vi "Config Load.vi"(8 "error in (no error)":errorcluster, 11 "Text":string) -> (0 "error out":errorcluster, 3 "Sections":T1(array[cluster]))   [LabVIEW 2018]
uses:
  <vilib>/regexp/Match Regular Expression.xnode
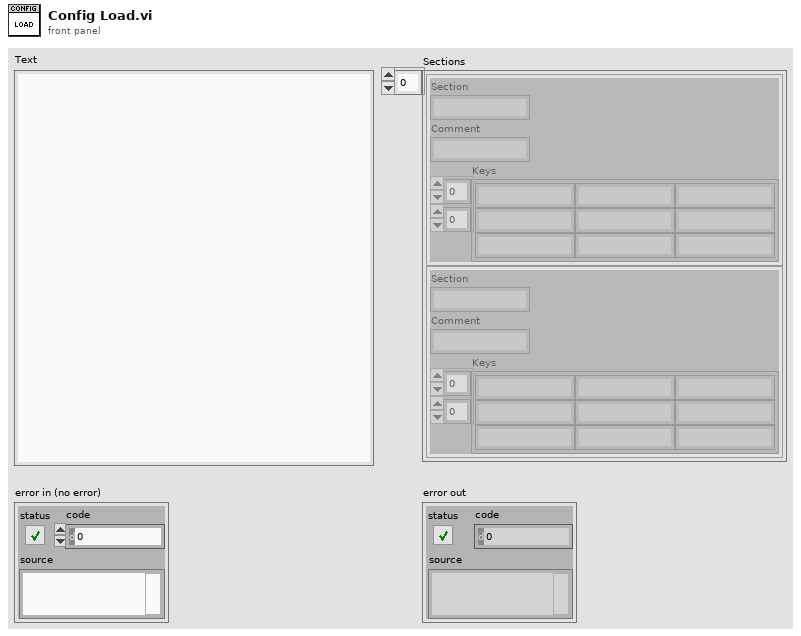
[diagram p1: front panel]
types:
  T1 = cluster{"Section":string, "Comment":string, "Keys":string[][]}[]
  T2 = cluster{"Section":string, "Comment":string, "Keys":string[][]}
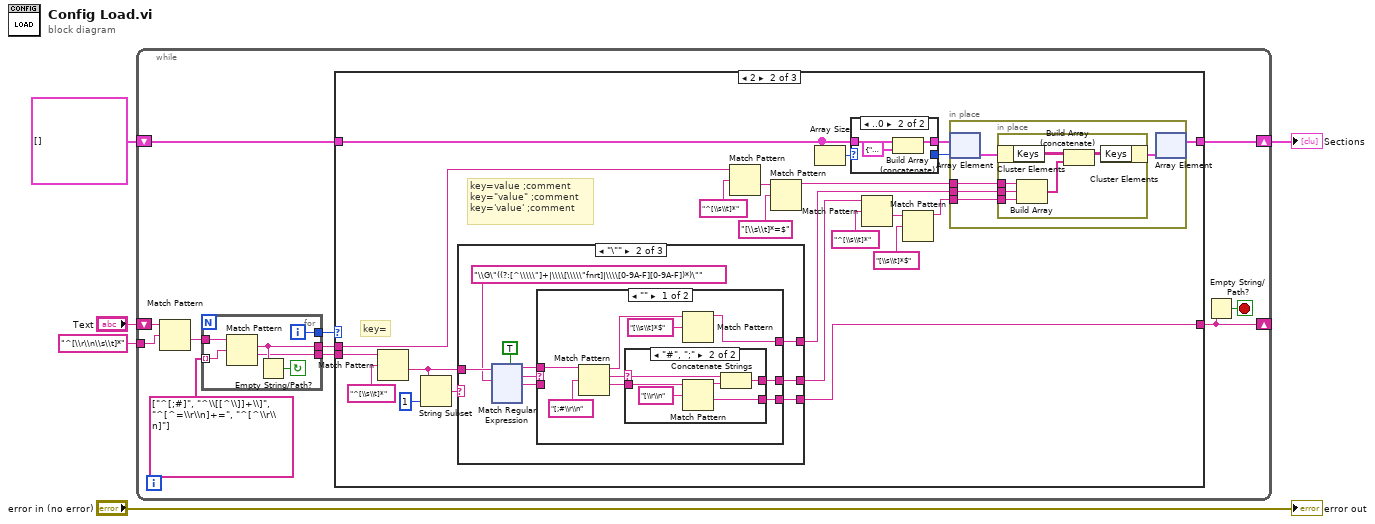
[diagram p0: block diagram]
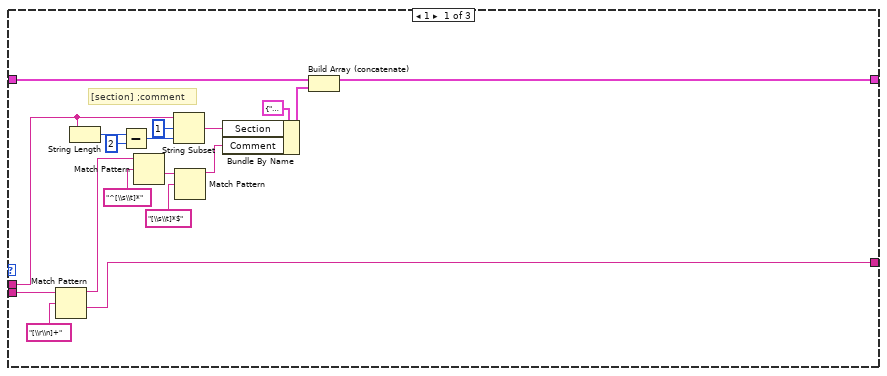
[diagram p2: hidden frame]
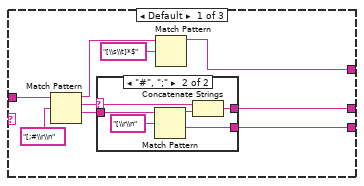
[diagram p3: hidden frame]
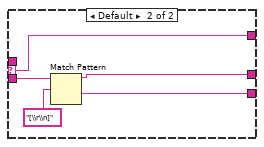
[diagram p6: hidden frame]
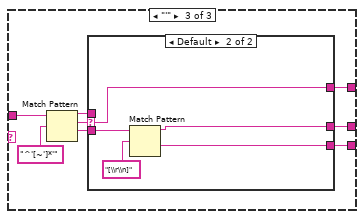
[diagram p7: hidden frame]
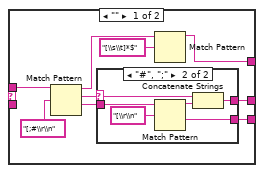
[diagram p8: hidden frame]
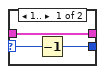
[diagram p10: hidden frame]
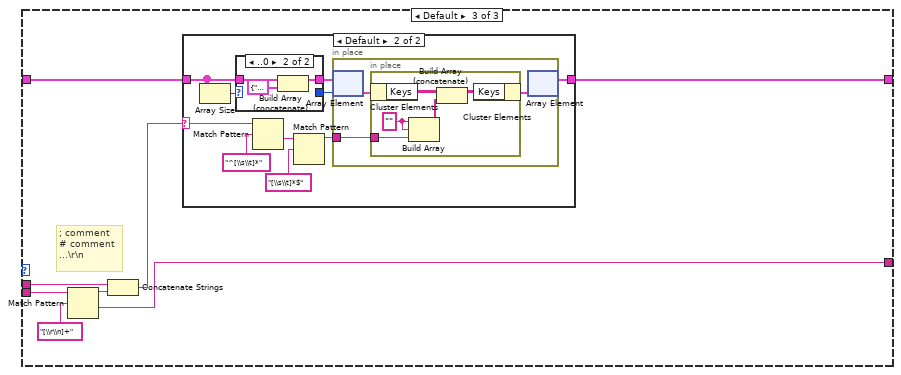
[diagram p11: hidden frame]
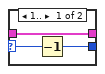
[diagram p13: hidden frame]
diagram:
  n1 = while {
    tunnel: "^[\\r\\n\\s\\t]*" ("regular expression") -> [w16]
    shift-right: [w9] -> _
    shift-left: "Text" -> [w15]
    shift-right: [w10] -> w1
    shift-left: T1 [] ("Sections") -> [w12]
    stop <- w8 stop-if-true
    n2 = Match Pattern(string=w15, regular expression=w16) -> (after substring=w14:string)  [unwired: 1 in, 3 out]
    n3 = for {
      tunnel: string[] ["^[;#]", "^\\[[^\\]]+\\]", "^[^=\\r\\n]+=", "^[^\\r\\n]"] -> [w304] mode=indexing
      tunnel: w14 -> [w303]
      tunnel: [w301] -> w7
      tunnel: [w300] -> w13
      tunnel: [w299] -> w11
      i -> [w300]
      stop <- w302 continue-if-true
      n4 = Match Pattern(string=w303, regular expression=w304) -> (match substring=w301:string, after substring=w299:string)  [unwired: 1 in, 2 out]
      n5 = Empty String/Path?(string/path=w301) -> (empty?=w302:bool)
    }
    n6 = case shown="2" w13 {
      tunnel: w12 -> [w21 w49 w273]
      tunnel: w11 -> [w18 w41 w269]
      tunnel: [w20 w48 w272] -> w10
      tunnel: [w17 w37 w268] -> w9
      tunnel: w7 -> [w19 w44 w266]
      frame 1 {
        # "[section] ;comment"
        n7 = Match Pattern(string=w18, regular expression="[\\r\\n]+") -> (before substring=w23:string, after substring=w17:string)  [unwired: 1 in, 2 out]
        n8 = String Length(string=w19) -> (length=w30:i32)
        n9 = Subtract(x=w30, y=2) -> (x-y=w28:i32)
        n10 = Match Pattern(string=w23, regular expression="^[\\s\\t]*") -> (after substring=w24:string)  [unwired: 1 in, 3 out]
        n11 = String Subset(string=w19, offset (0)=1, length (rest)=w28) -> (substring=w27:string)
        n12 = Match Pattern(string=w24, regular expression="[\\s\\t]*$") -> (before substring=w22:string)  [unwired: 1 in, 3 out]
        n13 = Bundle By Name(cluster=T2 {"Section"="", "Comment"="", "Keys"=[]} ("array"), "Section"=w27, "Comment"=w22) -> (w32:T2)
        n14 = Build Array (concatenate)(w21, w32) -> (w20:T1)
      }
      frame 2 {
        # "key=value ;comment\nkey=\"value\" ;comment\nkey='value' ;comment"
        # "key="
        n15 = Match Pattern(string=w41, regular expression="^[\\s\\t]*") -> (after substring=w38:string)  [unwired: 1 in, 3 out]
        n16 = String Subset(string=w38, length (rest)=1 ("length (rest)")) -> (substring=w39:string)  [unwired: 1 in]
        n17 = case shown="\"\\\"\"" w39 {
          tunnel: w38 -> [w64 w81 w224]
          tunnel: [w61 w74 w225] -> w37
          tunnel: [w60 w75 w226] -> w36
          tunnel: [w57 w78 w227] -> w35
          frame Default {
            n18 = Match Pattern(string=w64, regular expression="[;#\\r\\n") -> (before substring=w58:string, match substring=w62:string, after substring=w63:string)  [unwired: 1 in, 1 out]
            n19 = case shown="\"#\", \";\"" w62 {
              selector: w62 -> [_ w70]
              tunnel: w63 -> [w66 w71]
              tunnel: [w66 w68] -> w61
              tunnel: [_ w67] -> w60
              frame Default {
              }
              frame "#", ";" {
                n20 = Match Pattern(string=w71, regular expression="[\\r\\n") -> (before substring=w69:string, after substring=w68:string)  [unwired: 1 in, 2 out]
                n21 = Concatenate Strings(w70, w69) -> (w67:string)
              }
            }
            n22 = Match Pattern(string=w58, regular expression="[\\s\\t]*$") -> (before substring=w57:string)  [unwired: 1 in, 3 out]
          }
          frame "\"" {
            n23 = xnode "Match Regular Expression"("input string"=w81, "regular expression"="\\G\"((?:[^\\\\\"]+|\\\\[\\\\\"fnrt]|\\\\[0-9A-F][0-9A-F])*)\"", "multiline? (F)"=TRUE) -> ("before match"=w77:string, "whole match"=w79:string, "after match"=w76:string)  [unwired: 3 in, 2 out]
            n24 = case shown="\"\"" w79 {
              selector: w79 -> [_ w102]
              tunnel: [w82 w102] -> w78
              tunnel: w77 -> [w87 _]
              tunnel: w76 -> [_ w100]
              tunnel: [w86 w99] -> w75
              tunnel: [w85 w98] -> w74
              frame "" {
                n25 = Match Pattern(string=w87, regular expression="[;#\\r\\n") -> (before substring=w83:string, match substring=w88:string, after substring=w89:string)  [unwired: 1 in, 1 out]
                n26 = case shown="\"#\", \";\"" w88 {
                  selector: w88 -> [_ w95]
                  tunnel: w89 -> [w91 w96]
                  tunnel: [w91 w93] -> w85
                  tunnel: [_ w92] -> w86
                  frame Default {
                  }
                  frame "#", ";" {
                    n27 = Match Pattern(string=w96, regular expression="[\\r\\n") -> (before substring=w94:string, after substring=w93:string)  [unwired: 1 in, 2 out]
                    n28 = Concatenate Strings(w95, w94) -> (w92:string)
                  }
                }
                n29 = Match Pattern(string=w83, regular expression="[\\s\\t]*$") -> (before substring=w82:string)  [unwired: 1 in, 3 out]
              }
              frame Default {
                n30 = Match Pattern(string=w100, regular expression="[\\r\\n]") -> (before substring=w99:string, after substring=w98:string)  [unwired: 1 in, 2 out]
              }
            }
          }
          frame "'" {
            n31 = Match Pattern(string=w224, regular expression="^'[~']*'") -> (before substring=w223:string, match substring=w222:string, after substring=w221:string)  [unwired: 1 in, 1 out]
            n32 = case shown="Default" w222 {
              selector: w222 -> [_ w248]
              tunnel: [w228 w248] -> w227
              tunnel: w223 -> [w233 _]
              tunnel: w221 -> [_ w246]
              tunnel: [w232 w245] -> w226
              tunnel: [w231 w244] -> w225
              frame "" {
                n33 = Match Pattern(string=w233, regular expression="[;#\\r\\n") -> (before substring=w229:string, match substring=w234:string, after substring=w235:string)  [unwired: 1 in, 1 out]
                n34 = case shown="\"#\", \";\"" w234 {
                  selector: w234 -> [_ w241]
                  tunnel: w235 -> [w237 w242]
                  tunnel: [w237 w239] -> w231
                  tunnel: [_ w238] -> w232
                  frame Default {
                  }
                  frame "#", ";" {
                    n35 = Match Pattern(string=w242, regular expression="[\\r\\n") -> (before substring=w240:string, after substring=w239:string)  [unwired: 1 in, 2 out]
                    n36 = Concatenate Strings(w241, w240) -> (w238:string)
                  }
                }
                n37 = Match Pattern(string=w229, regular expression="[\\s\\t]*$") -> (before substring=w228:string)  [unwired: 1 in, 3 out]
              }
              frame Default {
                n38 = Match Pattern(string=w246, regular expression="[\\r\\n]") -> (before substring=w245:string, after substring=w244:string)  [unwired: 1 in, 2 out]
              }
            }
          }
        }
        n39 = Match Pattern(string=w44, regular expression="^[\\s\\t]*") -> (after substring=w47:string)  [unwired: 1 in, 3 out]
        n40 = Match Pattern(string=w47, regular expression="[\\s\\t]*=$") -> (before substring=w43:string)  [unwired: 1 in, 3 out]
        n41 = Array Size(array=w49) -> (size(s)=w56:i32)
        n42 = case shown="..0" w56 {
          selector: w56 -> [w261 _]
          tunnel: w49 -> [w262 w265]
          tunnel: [w262 w264] -> w55
          tunnel: [w260 _] -> w54
          frame 1.. {
            n43 = Decrement(x=w261) -> (x-1=w260:i32)
          }
          frame ..0 {
            n44 = Build Array (concatenate)(w265, T2 {"Section"="", "Comment"="", "Keys"=[]} ("array")) -> (w264:T1)
          }
        }
        n45 = Match Pattern(string=w36, regular expression="^[\\s\\t]*") -> (after substring=w51:string)  [unwired: 1 in, 3 out]
        n46 = Match Pattern(string=w51, regular expression="[\\s\\t]*$") -> (before substring=w50:string)  [unwired: 1 in, 3 out]
        n47 = in-place {
          in-place-border: w50 -> [w251]
          in-place-border: w43 -> [w250]
          in-place-border: w35 -> [w249]
          n48 = in-place-array #1(w55, w54) -> (w253:T2)
          n49 = in-place {
            in-place-border: w251 -> [w256]
            in-place-border: w250 -> [w255]
            in-place-border: w249 -> [w254]
            n50 = in-place-cluster #2(w253) -> ("Keys"=w259:string[][])
            n51 = Build Array(w255, w254, w256) -> (w257:string[])
            n52 = Build Array (concatenate)(w259, w257) -> (w258:string[][])
            n53 = in-place-cluster #2("Keys"=w258) -> (w252:T2)
          }
          n54 = in-place-array #1(w252) -> (w48:T1)  [unwired: 1 out]
        }
      }
      frame Default {
        # "; comment\n# comment\n...\\r\\n"
        n55 = Match Pattern(string=w269, regular expression="[\\r\\n]+") -> (before substring=w270:string, after substring=w268:string)  [unwired: 1 in, 2 out]
        n56 = Concatenate Strings(w266, w270) -> (w267:string)
        n57 = case shown="Default" w267 {
          selector: w267 -> [_ w275]
          tunnel: w273 -> [w274 w277]
          tunnel: [w274 w276] -> w272
          frame "" {
          }
          frame Default {
            n58 = Array Size(array=w277) -> (size(s)=w284:i32)
            n59 = case shown="..0" w284 {
              selector: w284 -> [w286 _]
              tunnel: w277 -> [w287 w290]
              tunnel: [w287 w289] -> w283
              tunnel: [w285 _] -> w282
              frame 1.. {
                n60 = Decrement(x=w286) -> (x-1=w285:i32)
              }
              frame ..0 {
                n61 = Build Array (concatenate)(w290, T2 {"Section"="", "Comment"="", "Keys"=[]} ("array")) -> (w289:T1)
              }
            }
            n62 = Match Pattern(string=w275, regular expression="^[\\s\\t]*") -> (after substring=w279:string)  [unwired: 1 in, 3 out]
            n63 = Match Pattern(string=w279, regular expression="[\\s\\t]*$") -> (before substring=w278:string)  [unwired: 1 in, 3 out]
            n64 = in-place {
              in-place-border: w278 -> [w291]
              n65 = in-place-array #3(w283, w282) -> (w293:T2)
              n66 = in-place {
                in-place-border: w291 -> [w294]
                w296 = ""
                n67 = in-place-cluster #4(w293) -> ("Keys"=w298:string[][])
                n68 = Build Array(w296, w296, w294) -> (w295:string[])
                n69 = Build Array (concatenate)(w298, w295) -> (w297:string[][])
                n70 = in-place-cluster #4("Keys"=w297) -> (w292:T2)
              }
              n71 = in-place-array #3(w292) -> (w276:T1)  [unwired: 1 out]
            }
          }
        }
      }
    }
    n72 = Empty String/Path?(string/path=w9) -> (empty?=w8:bool)
  }
  "Sections" <- w1
  "error out" <- "error in (no error)"
